vi "Parse Tree Labels.vi"(8 "error out":errorcluster, 9 "Specified Channel Ref List":T1[](array[typedef]) format="%.0x", 10 "Label Refs":T1[](array[typedef]) format="%.0x", 11 "Custom Device Ref":T1 format="%.0x") -> (0 "error out":errorcluster, 3 "Label data":T2[](array[typedef]) {"Word"."Param Setting"."Num Bits" min=1 max=32; "Word"."Param Setting"."Start Bit" min=8 max=31; "Label" format="%.0o"})   [LabVIEW 2016, in "Ballard Arinc-429 System Explorer.lvlib"]
uses:
  System Explorer/Ballard Arinc-429 System Explorer.lvlib
  <vilib>/NI Veristand/Custom Device API/Custom Device API.lvlib
  Shared/Controls and Global/Global.vi
  Shared/Ballard Arinc-429 Shared.lvlib
  <vilib>/NI Veristand/Custom Device API/Get Item Property (U32).vi
  <vilib>/NI Veristand/Custom Device Tools/Custom Device Utility Library/Custom Device Utility Library.lvlib
  Shared/Controls and Global/TransferType.ctl
  Shared/Controls and Global/Start Bit.ctl
  Shared/Controls and Global/Number of Bits.ctl
  RT Controls/RT Param Setting.ctl
  Ballard Arinc-429 Engine.lvlib
  RT Controls/RT Word Settings.ctl
  Shared/Controls and Global/Label.ctl
  Shared/Controls and Global/transferPeriod.ctl
  RT Controls/RT Label Settings.ctl
  <vilib>/NI Veristand/Custom Device Tools/Custom Device Utility Library/NI VeriStand - Search for Item by GUID.vi
  <vilib>/NI Veristand/Custom Device API/Get Item Property (String).vi
  <vilib>/NI Veristand/Custom Device API/Custom Device Item Ref.ctl
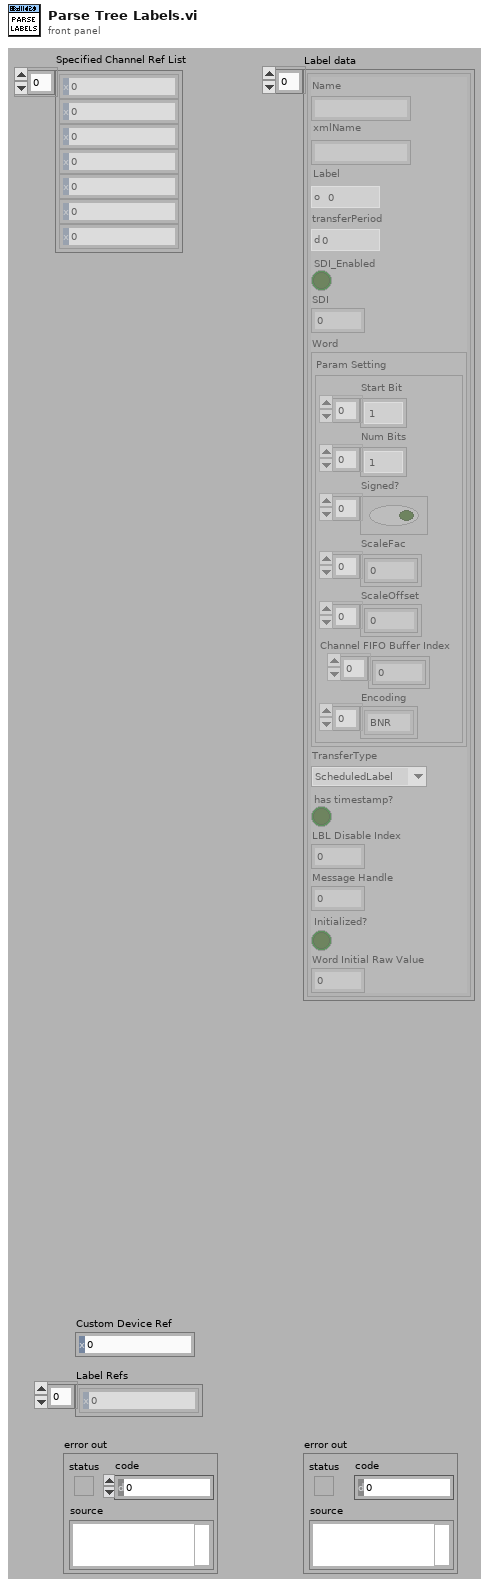
[diagram p1: front panel]
types:
  T1 = typedef "Custom Device API.lvlib/Custom Device Item Ref.ctl" = u64
  T2 = typedef "Ballard Arinc-429 Engine.lvlib/RT Label Settings.ctl" = cluster{"Name":string, "xmlName":string, "Label":T3, "transferPeriod":T4, "SDI_Enabled":bool, "SDI":u8, "Word":T5, "TransferType":T9, "has timestamp?":bool, "LBL Disable Index":i32, "Message Handle":u64, "Initialized?":bool, "Word Initial Raw Value":u32}
  T3 = typedef "Ballard Arinc-429 Shared.lvlib/Label.ctl" = u8
  T4 = typedef "Ballard Arinc-429 Shared.lvlib/transferPeriod.ctl" = u32
  T5 = typedef "Ballard Arinc-429 Engine.lvlib/RT Word Settings.ctl" = cluster{"Param Setting":T6}
  T6 = typedef "Ballard Arinc-429 Engine.lvlib/RT Param Setting.ctl" = cluster{"Start Bit":T7[], "Num Bits":T8[], "Signed?":bool[], "ScaleFac":dbl[], "ScaleOffset":dbl[], "Channel FIFO Buffer Index":i32[], "Encoding":enum16{"BNR", "BCD", "Discrete"}[]}
  T7 = typedef "Ballard Arinc-429 Shared.lvlib/Start Bit.ctl" = i32
  T8 = typedef "Ballard Arinc-429 Shared.lvlib/Number of Bits.ctl" = i32
  T9 = typedef "Ballard Arinc-429 Shared.lvlib/TransferType.ctl" = enum16{"ScheduledLabel", "Acyclic", "Block", "Strobe"}
  T10 = typedef "Custom Device API.lvlib/Custom Device Item Info.ctl" = cluster{"Name":string, "Is Channel":bool, "GUID":string, "Is Waveform":bool}
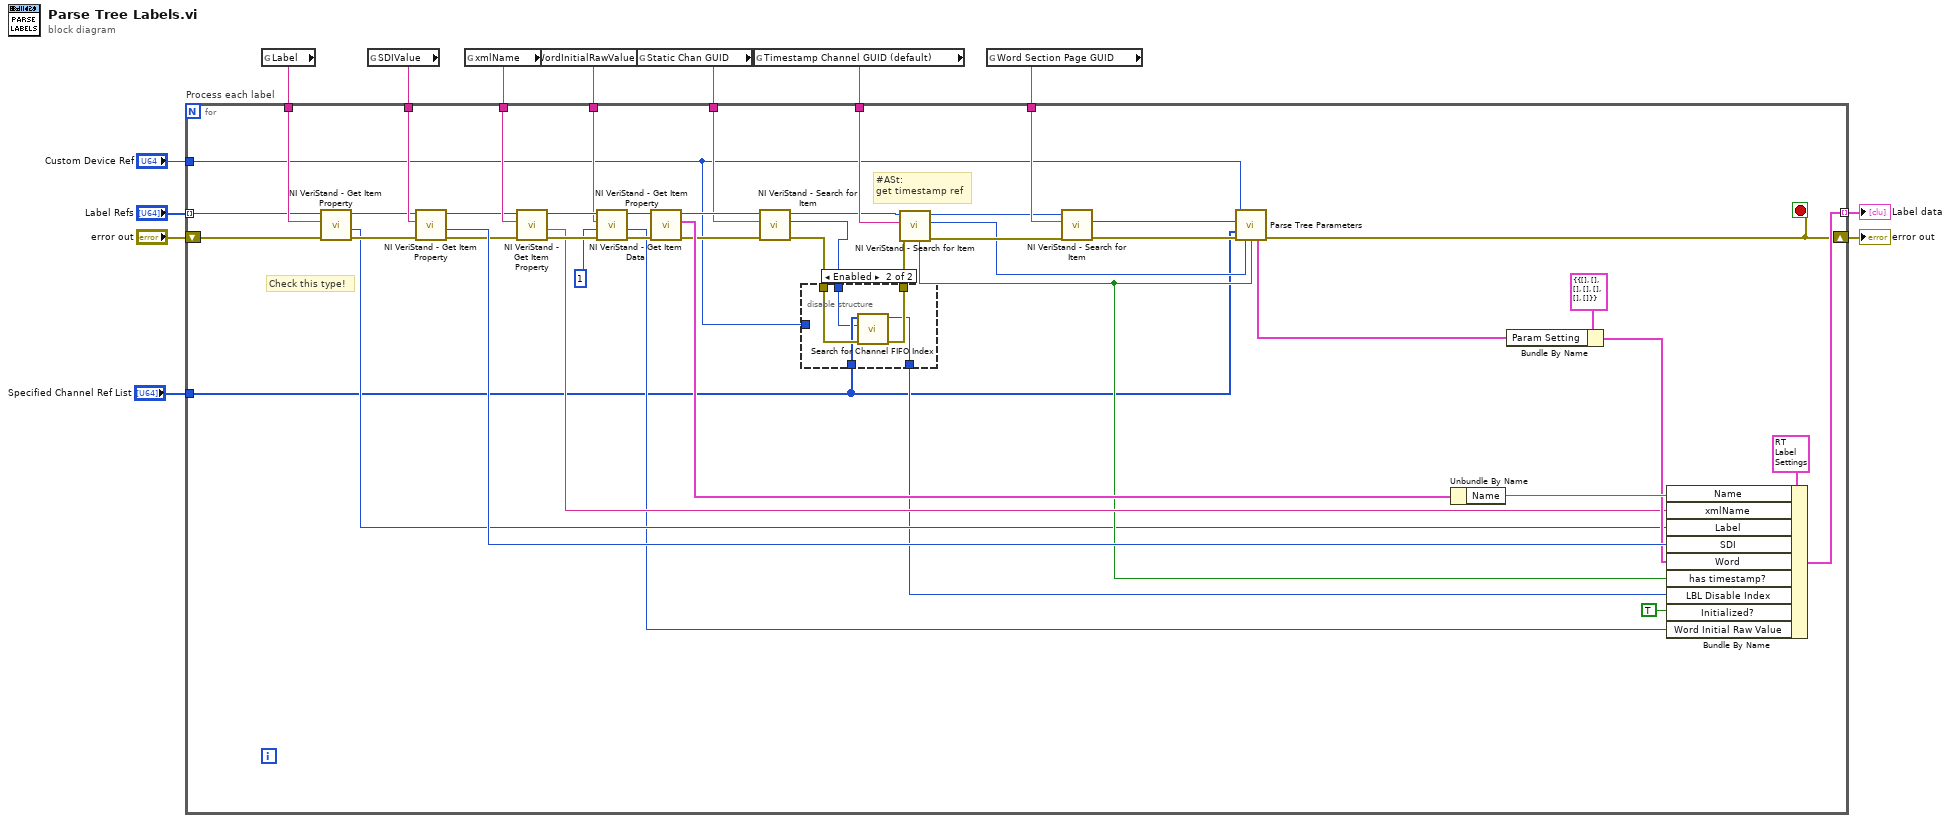
[diagram p0: block diagram]
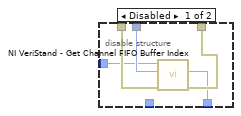
[diagram p2: hidden frame]
diagram:
  n1 = global read "Global.vi" "Label"() -> (w3:string)
  n2 = global read "Global.vi" "SDIValue"() -> (w9:string)
  n3 = global read "Global.vi" "xmlName"() -> (w8:string)
  n4 = global read "Global.vi" "WordInitialRawValue"() -> (w7:string)
  n5 = global read "Global.vi" "Static Chan GUID"() -> (w2:string)
  n6 = global read "Global.vi" "Timestamp Channel GUID (default)"() -> (w5:string)
  n7 = global read "Global.vi" "Word Section Page GUID"() -> (w6:string)
  n8 = for "Process each label" {
    tunnel: "Label Refs" -> [w35] mode=indexing
    shift-right: [w39] -> w10
    shift-left: "error out" -> [w38]
    tunnel: "Custom Device Ref" -> [w20]
    tunnel: w9 -> [w59]
    tunnel: w8 -> [w58]
    tunnel: w7 -> [w54]
    tunnel: w6 -> [w51]
    tunnel: w5 -> [w47]
    tunnel: [w43] -> w4 mode=indexing
    tunnel: w3 -> [w36]
    tunnel: w2 -> [w28]
    tunnel: "Specified Channel Ref List" -> [w14]
    stop <- w39 stop-if-true
    # "Check this type!"
    # "#ASt:\nget timestamp ref"
    n9 = call-poly <vilib>:"NI VeriStand - Get Item Property.vi"("error in (no error)"=w38, "Property Name"=w36, "Item Ref in"=w35) -> ("error out"=w37:errorcluster, "Value"=w25:u32, "Item Ref out"=w34:T1)  [unwired: 5 in, 1 out]
    n10 = call-poly <vilib>:"NI VeriStand - Get Item Property.vi"("error in (no error)"=w37, "Property Name"=w59, "Item Ref in"=w34) -> ("error out"=w26:errorcluster, "Value"=w45:u32, "Item Ref out"=w27:T1)  [unwired: 5 in, 1 out]
    n11 = call-poly <vilib>:"NI VeriStand - Get Item Property.vi"("error in (no error)"=w26, "Property Name"=w58, "Item Ref in"=w27) -> ("error out"=w57:errorcluster, "Value"=w40:string, "Item Ref out"=w55:T1)  [unwired: 5 in, 1 out]
    n12 = call-poly <vilib>:"NI VeriStand - Get Item Property.vi"("error in (no error)"=w57, "Default Value"=u32 1, "Property Name"=w54, "Item Ref in"=w55) -> ("error out"=w56:errorcluster, "Value"=w15:u32, "Item Ref out"=w53:T1)  [unwired: 4 in, 1 out]
    n13 = call <vilib>:"NI VeriStand - Get Item Data.vi"("error in (no error)"=w56, "Item Ref in"=w53) -> ("error out"=w30:errorcluster, "Item Info"=w33:T10, "Item Ref out"=w29:T1)  [unwired: 6 in, 1 out]
    n14 = call-poly <vilib>:"NI VeriStand - Search for Item.vi"("error in"=w30, "Item GUID"=w28, "Section Ref in"=w29) -> ("error out"=w24:errorcluster, "Item Ref"=w22:T1, "Section Ref out"=w21:T1)  [unwired: 5 in, 1 out]
    n15 = disable-structure shown="Enabled" {
      disable-tunnel: w24 -> [w64 w69]
      disable-tunnel: [w63 w68] -> w23
      disable-tunnel: w22 -> [w62 w66]
      disable-tunnel: w20 -> [w61 _]
      disable-tunnel: [w60 w65] -> w19
      disable-tunnel: w14 -> [_ w67]
      frame Disabled {
        n16 = call <vilib>:"NI VeriStand - Get Channel FIFO Buffer Index.vi"("error in"=w64, "Channel Ref"=w62, "Device Ref in"=w61) -> ("error out"=w63:errorcluster, "Channel FIFO Buffer Index"=w60:i32)  [unwired: 4 in, 3 out]
      }
      frame Enabled {
        n17 = call "Search for Channel FIFO Index.vi"("error in (no error)"=w69, "Item Ref"=w66, "Specified Channel Ref List"=w67) -> ("error out"=w68:errorcluster, "index of element"=w65:i32)  [unwired: 7 in]
      }
    }
    n18 = call-poly <vilib>:"NI VeriStand - Search for Item.vi"("error in"=w23, "Item GUID"=w47, "Section Ref in"=w21) -> ("error out"=w49:errorcluster, "Item Ref"=w46:T1, "Section Ref out"=w48:T1, "Found"=w31:bool)  [unwired: 5 in]
    n19 = call-poly <vilib>:"NI VeriStand - Search for Item.vi"("error in"=w49, "Item GUID"=w51, "Section Ref in"=w48) -> ("error out"=w52:errorcluster, "Item Ref"=w32:T1)  [unwired: 5 in, 2 out]
    n20 = call "Parse Tree Parameters.vi"("Custom Device Ref"=w20, "Item Ref in"=w32, "Specified Channel Ref List"=w14, "error in"=w52, "Timestamp Ref"=w46, "Timestamp?"=w31) -> ("Parameter Driver Data"=w16:T6, "error out"=w39:errorcluster)  [unwired: 7 in, 1 out]
    n21 = Unbundle By Name(w33) -> ("Name"=w44:string)
    n22 = Bundle By Name(cluster=T5 {"Param Setting"={"Start Bit"=[], "Num Bits"=[], "Signed?"=[], "ScaleFac"=[], "ScaleOffset"=[], "Channel FIFO Buffer Index"=[], "Encoding"=[]}} ("Word"), "Param Setting"=w16) -> (w41:T5)
    n23 = Bundle By Name(cluster=T2 {"Name"="", "xmlName"="", "Label"=0, "transferPeriod"=0, "SDI_Enabled"=FALSE, "SDI"=0, "Word"={"Param Setting"={"Start Bit"=[], "Num Bits"=[], "Signed?"=[], "ScaleFac"=[], "ScaleOffset"=[], "Channel FIFO Buffer Index"=[], "Encoding"=[]}}, "TransferType"=enum."ScheduledLabel", "has timestamp?"=FALSE, "LBL Disable Index"=0, "Message Handle"=0, "Initialized?"=FALSE, "Word Initial Raw Value"=0} ("Label Settings"), "Name"=w44, "xmlName"=w40, "Label"=w25, "SDI"=w45, "Word"=w41, "has timestamp?"=w31, "LBL Disable Index"=w19, "Initialized?"=TRUE, "Word Initial Raw Value"=w15) -> (w43:T2)
  }
  "Label data" <- w4
  "error out" <- w10
